vi "HKEYS.vi"(8 "error in (no error)":errorcluster, 10 "key":string, 11 "Redis Client in":refnum<class "Redis Client.lvclass">) -> (0 "error out":errorcluster, 2 "fields":variant[](array[variant]), 3 "Redis Client out":refnum<class "Redis Client.lvclass">)   [LabVIEW 2019, in "Redis Client for LabVIEW.lvlib" / "Redis Client.lvclass"]
uses:
  Redis Client.lvclass
  lib/RESP3-for-LabVIEW/RESP3/subVIs/RESP3 Make String Base.vi
  lib/RESP3-for-LabVIEW/RESP3/types/RESP3 data type attribute.vi
  lib/RESP3-for-LabVIEW/RESP3/RESP3.lvlib
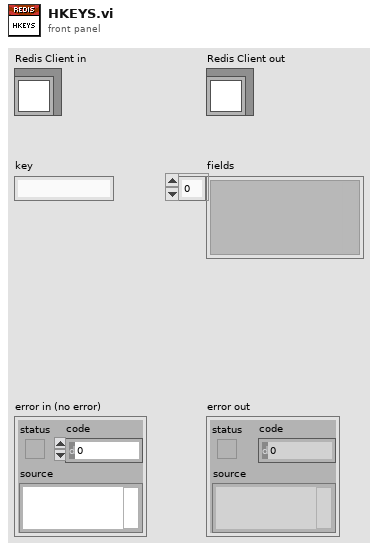
[diagram p1: front panel]
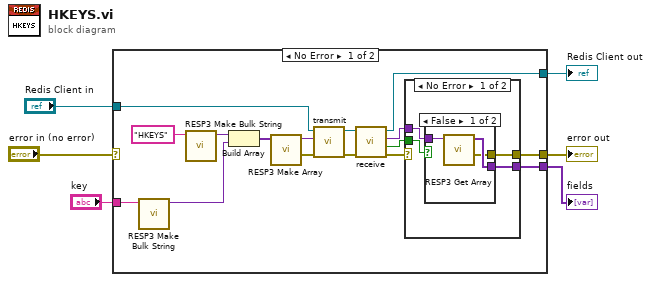
[diagram p0: block diagram]
diagram:
  n1 = case shown="No Error" "error in (no error)" {
    selector: "error in (no error)" -> [_ w32]
    tunnel: [w10 w32] -> w5
    tunnel: "Redis Client in" -> [w22 w31]
    tunnel: [w19 w31] -> w3
    tunnel: "key" -> [w16 _]
    tunnel: [w7 _] -> w1
    frame No Error {
      n2 = call "RESP3 Make Bulk String.vi"("String"=w16) -> ("RESP3 Value out"=w14:variant)  [unwired: 9 in, 1 out]
      n3 = call "RESP3 Make Bulk String.vi"("String"="HKEYS" ("string in")) -> ("RESP3 Value out"=w15:variant)  [unwired: 9 in, 1 out]
      n4 = Build Array(w15, w14) -> (w21:variant[])
      n5 = call "RESP3 Make Array.vi"("RESP3 Values in"=w21) -> ("error out"=w12:errorcluster, "RESP3 Value out"=w13:variant)  [unwired: 9 in]
      n6 = call-dynamic "transmit.vi"("error in (no error)"=w12, "RESP3 Value"=w13, "Redis Client in"=w22) -> ("error out"=w18:errorcluster, "Redis Client out"=w20:refnum<class "Redis Client.lvclass">)  [unwired: 7 in]
      n7 = call-dynamic "receive.vi"("error in (no error)"=w18, "Redis Client in"=w20) -> ("error out"=w9:errorcluster, "timed out?"=w8:bool, "RESP3 Value"=w11:variant, "Redis Client out"=w19:refnum<class "Redis Client.lvclass">)  [unwired: 6 in]
      n8 = case shown="No Error" w9 {
        selector: w9 -> [_ w30]
        tunnel: w11 -> [w26 _]
        tunnel: [w23 w30] -> w10
        tunnel: w8 -> [w25 _]
        tunnel: [w24 _] -> w7
        frame No Error {
          n9 = case shown="False" w25 {
            tunnel: w26 -> [w29 _]
            tunnel: [w28 _] -> w24
            tunnel: [w27 _] -> w23
            frame False {
              n10 = call "RESP3 Get Array.vi"("RESP3 Value in"=w29) -> ("error out"=w27:errorcluster, "RESP3 Values out"=w28:variant[])  [unwired: 7 in, 2 out]
            }
            frame True {
            }
          }
        }
        frame Error {
        }
      }
    }
    frame Error {
    }
  }
  "error out" <- w5
  "Redis Client out" <- w3
  "fields" <- w1
